vi "Pin Position Display.vi"(8 "error in (no error)":errorcluster) -> (0 "error out":errorcluster)   [LabVIEW 2013]
uses:
  Data Access Objects/Metadata/LBCB Number.ctl
  Data Access Objects/Metadata/Persistant DAO Actions.ctl
panel:
  in  "Axis Messages":string[](array[string])=["Positive X is in the direction of LBCB1 X actuators EXTENSION", "Positive X is in the direction of LBCB1 X actuators RETRACTION"]
  in  "LBCB Number":T1
  in  "Pin Messages":string[](array[string])=[" pin locations for X actuators are NEGATIVE on the X axis", " pin locations for X actuators are POSITVE on the X axis"]
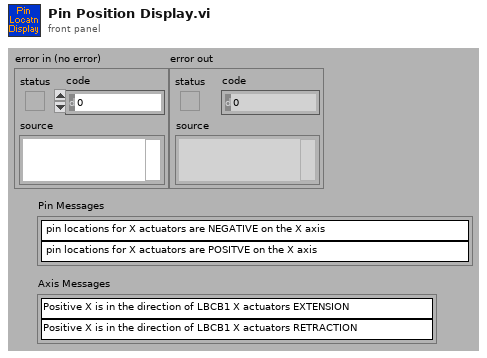
[diagram p1: front panel]
types:
  T1 = typedef "LBCB Number.ctl" = enum16{"LBCB1", "LBCB2"}
  T2 = typedef "Persistant DAO Actions.ctl" = enum16{"Init", "Get", "Set", "Load", "Save"}
  T3 = typedef "Pin Positions.ctl" = cluster{"Pin Positions":dbl[][], "Row Labels":string[]}
  T4 = typedef "Number Of LBCBs.ctl" = enum16{"1", "2"}
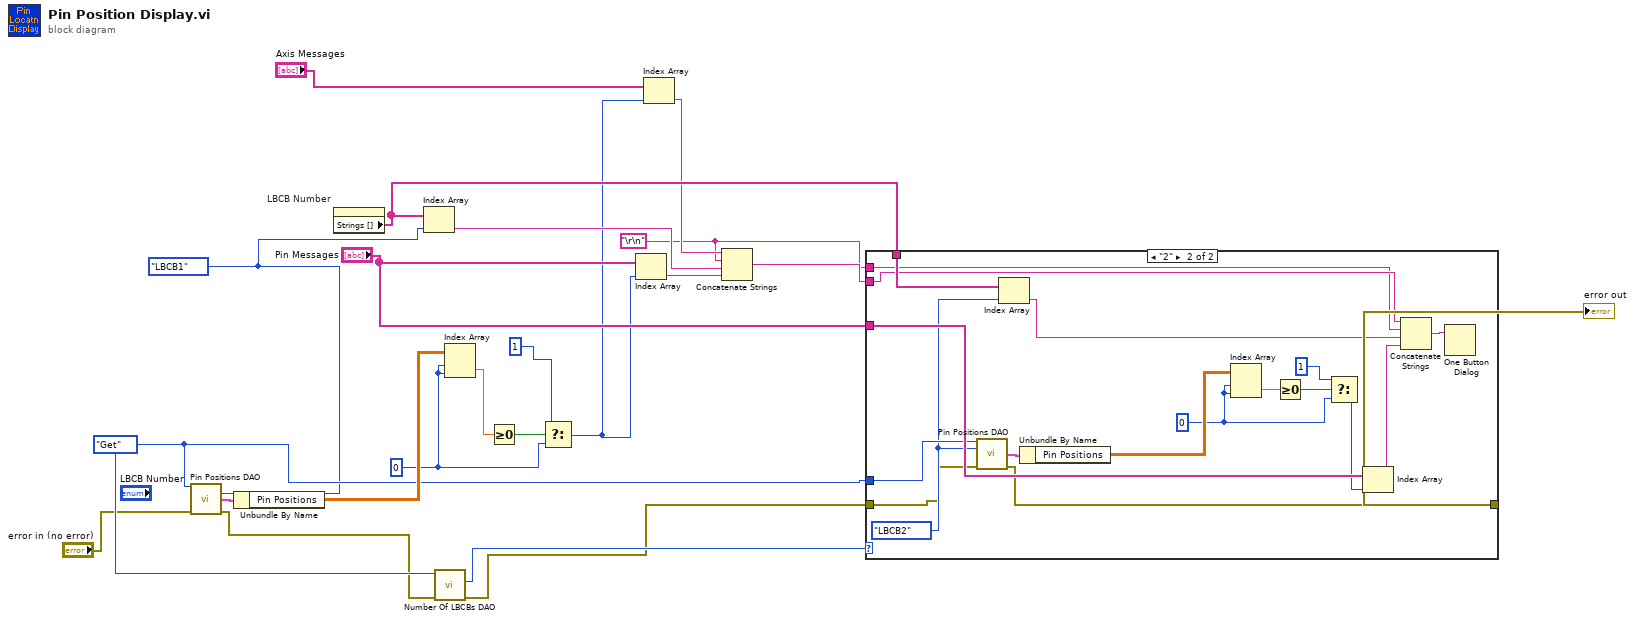
[diagram p0: block diagram]
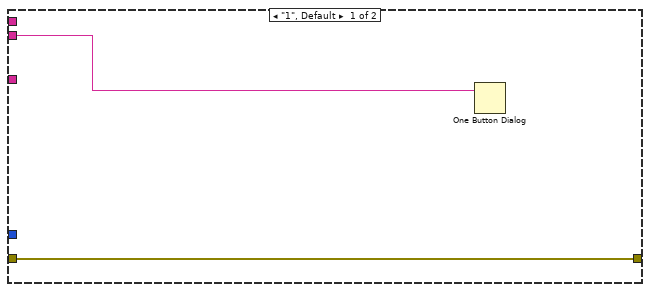
[diagram p2: hidden frame]
diagram:
  w1 = 0 ("index (row)")
  w11 = "\r\n"
  w8 = LBCB_Number."LBCB1" ("LBCB Number")
  w9 = Persistant_DAO_Actions."Get" ("Actions")
  n1 = call "Pin Positions DAO.vi"("LBCB Settings Actions"=w9, "LBCB Number"=w8, "error in (no error)"="error in (no error)") -> ("LBCB Pins Output"=w10:T3, "error out"=w6:errorcluster)  [unwired: 10 in, 1 out]
  n2 = Unbundle By Name(w10) -> ("Pin Positions"=w14:dbl[][])
  n3 = property on="LBCB Number" class="Enum (strict)"() -> ("Strings []"=w19:string[])  [unwired: 2 in, 2 out]
  n4 = Index Array(array=w19, index=w8) -> (element=w20:string)
  n5 = call "Number Of LBCBs DAO.vi"("error in (no error)"=w6, "Actions"=w9) -> ("error out"=w16:errorcluster, "Number of\nLBCBs Out"=w21:T4)  [unwired: 6 in, 2 out]
  n6 = Index Array(array=w14, index (row)=w1, index (col)=w1) -> (element=w5:dbl)
  n7 = Greater Or Equal To 0?(x=w5) -> (x >= 0?=w4:bool)
  n8 = Select(t=1, s=w4, f=w1) -> (s? t:f=w3:i32)
  n9 = Index Array(array="Pin Messages", index=w3) -> (element=w22:string)
  n10 = Index Array(array="Axis Messages", index=w3) -> (element=w12:string)
  n11 = Concatenate Strings(w12, w11, w20, w22) -> (w13:string)
  n12 = case shown="\"2\"" w21 {
    tunnel: w9 -> [_ w29]
    tunnel: w19 -> [_ w39]
    tunnel: "Pin Messages" -> [_ w38]
    tunnel: [w24 w26] -> w17
    tunnel: w16 -> [w24 w27]
    tunnel: w13 -> [w23 w37]
    tunnel: w11 -> [_ w36]
    frame "1", Default {
      n13 = One Button Dialog(message=w23) -> ()  [unwired: 1 in, 1 out]
    }
    frame "2" {
      w30 = 0 ("index (row)")
      w28 = LBCB_Number."LBCB2" ("LBCB Number")
      n14 = call "Pin Positions DAO.vi"("LBCB Settings Actions"=w29, "LBCB Number"=w28, "error in (no error)"=w27) -> ("LBCB Pins Output"=w34:T3, "error out"=w26:errorcluster)  [unwired: 10 in, 1 out]
      n15 = Index Array(array=w39, index=w28) -> (element=w42:string)
      n16 = Unbundle By Name(w34) -> ("Pin Positions"=w35:dbl[][])
      n17 = Index Array(array=w35, index (row)=w30, index (col)=w30) -> (element=w33:dbl)
      n18 = Greater Or Equal To 0?(x=w33) -> (x >= 0?=w32:bool)
      n19 = Select(t=1, s=w32, f=w30) -> (s? t:f=w25:i32)
      n20 = Index Array(array=w38, index=w25) -> (element=w41:string)
      n21 = Concatenate Strings(w37, w36, w42, w41) -> (w40:string)
      n22 = One Button Dialog(message=w40) -> ()  [unwired: 1 in, 1 out]
    }
  }
  "error out" <- w17
